vi "ParallelDHT22andBMP180.vi"() -> ()   [LabVIEW 2016]
uses:
  <vilib>/userdefined/High Color/nirio_resource_hc.ctl
  <vilib>/FPGAPlugInAG/myRIO-1900/niLvFpga_Open_myRIO-1900.vi
  <vilib>/FPGAPlugInAG/myRIO-1900/niLvFpga_Run_myRIO-1900.vi
  <vilib>/Utility/error.llb/Error Cluster From Error Code.vi
  <vilib>/rvi/errors/niLvFpgaAdjustHostInterfaceError.vi
  <vilib>/FPGAPlugInAG/myRIO-1900/niLvFpga_Close_myRIO-1900.vi
  <vilib>/rvi/interface/nirviOpenFPGA/nirviOpenFPGA.xnode
  FPGA Bitfiles/WeatherStationPr_FPGATarget_HumiditySensorIn_HuBObqjwKeQ.lvbitx
  <vilib>/rvi/interface/nirviMethod/nirviMethod.xnode
  <vilib>/rvi/interface/nirviReadWriteControl/nirviReadWriteControl.xnode
  <vilib>/rvi/interface/nirviCloseFPGA/nirviCloseFPGA.xnode
  NiFpgaLv.dll
panel:
  in  "stop":bool
  out "Device_ID 2":u8[](array[numeric]) format="%.0x"
  out "READ MSB CAL_PARAM 2":u8[][](array[numeric]) format="%.0x"
  out "READ LSB CAL_PARAM 2":u8[][](array[numeric]) format="%.0x"
  out "Array 3":i16[][](array[numeric])
  out "UP_Value":u16[](array[numeric])
  out "UT_Value 2":u16[](array[numeric])
  out "Temperature(°C)":dbl
  out "Pressure in Pa.":dbl
  out "Waveform Chart Temperature":dbl(graph)
  out "Waveform Chart Presssure":dbl(graph)
  out "error out 2":errorcluster
  out "Waveform Chart":cluster{dbl, dbl}(graph)
  out "Temperature (°C)":fxp<+,16,7> format="%#_3g"
  out "Humidity (%)":fxp<+/-,18,8> format="%#_3g"
  out "Humidity sensor Communication":errorcluster
  out "FPGA Error":errorcluster
  in  "stop 2":bool
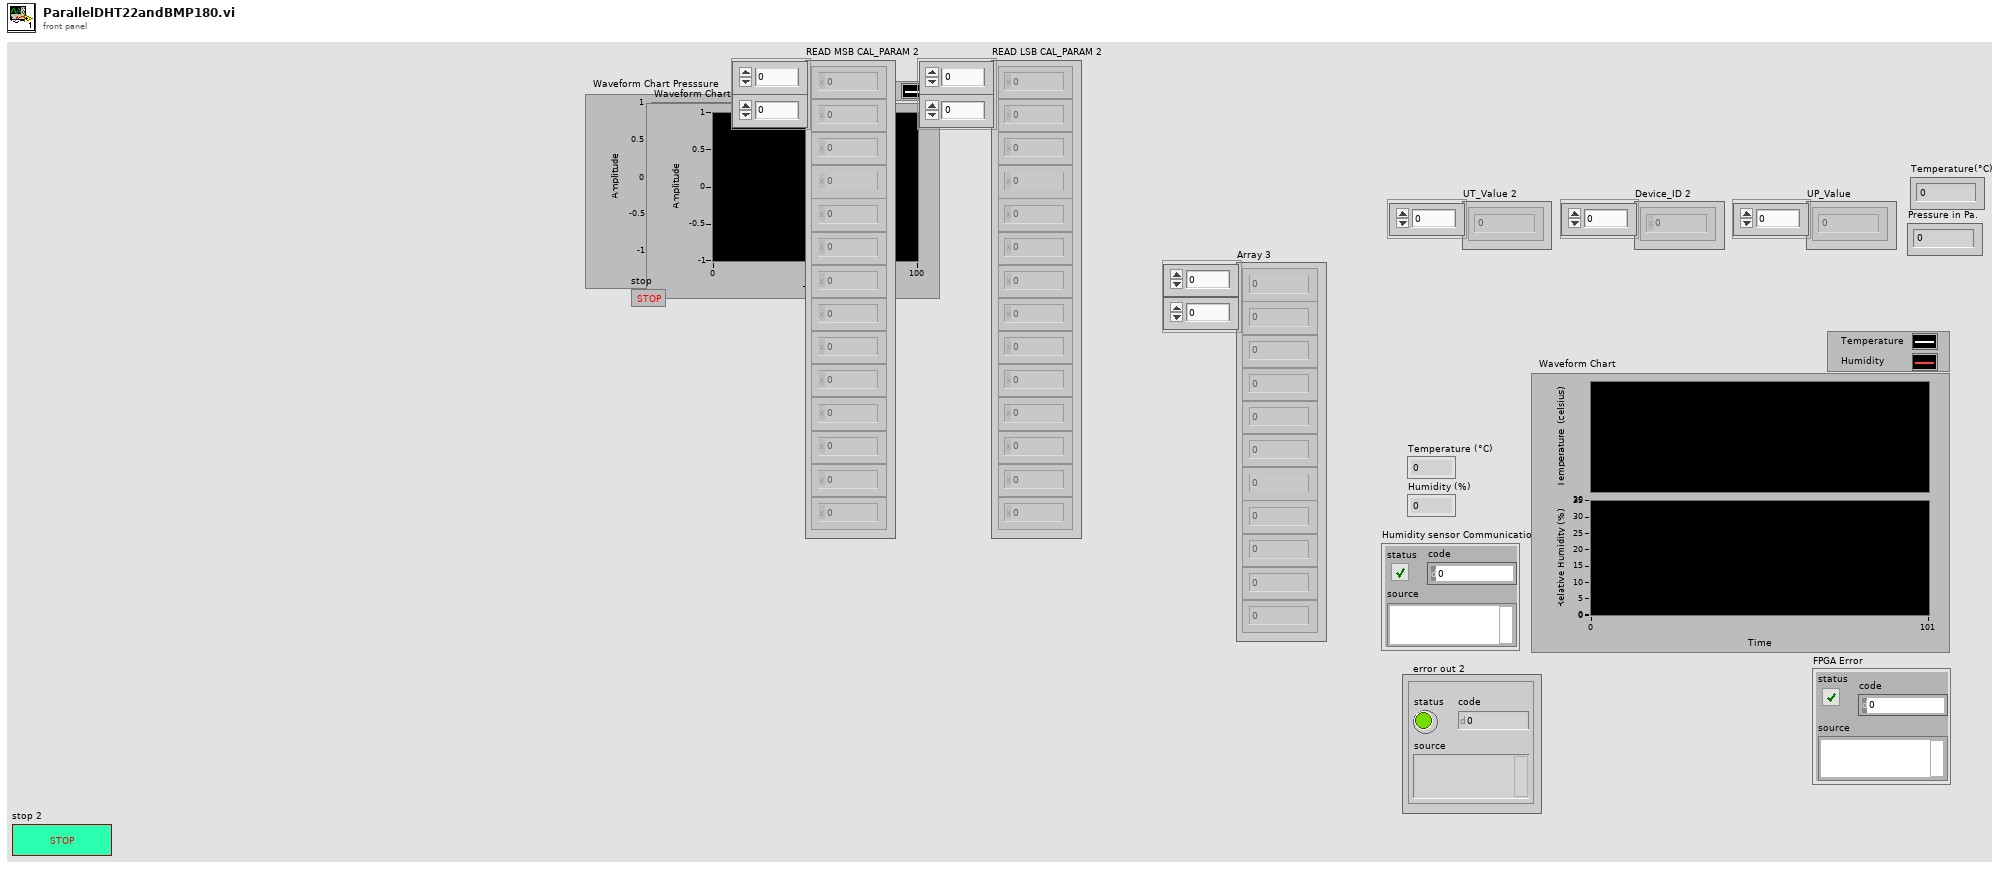
[diagram p1: front panel]
types:
  T1 = typedef "nirio_resource_hc.ctl" = tag
  T2 = cluster{"Temperature (°C)":fxp<+,16,7>, "Humidity (%)":fxp<+/-,18,8>}
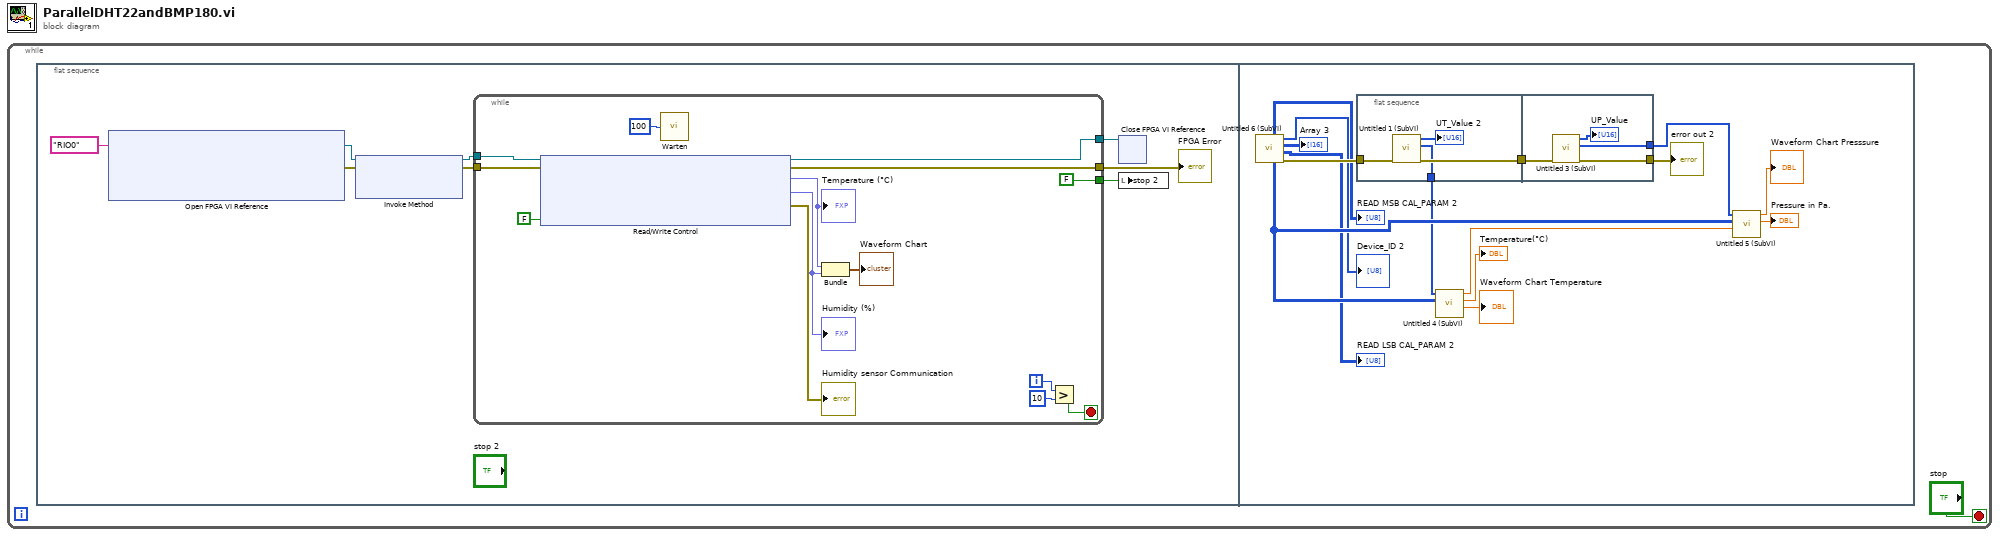
[diagram p0: block diagram]
diagram:
  n1 = while {
    stop <- "stop" stop-if-true
    n2 = flat-sequence {
      frame #0 {
        n3 = xnode "Open FPGA VI Reference"("resource name"=T1 "RIO0") -> ("FPGA VI Reference Out"=w6:refnum<k20>, "error out"=w5:errorcluster)  [unwired: 1 in]
        n4 = xnode "Invoke Method"("FPGA VI Reference In"=w6, "error in"=w5) -> ("FPGA VI Reference Out"=w4:refnum<k20>, "error out"=w3:errorcluster)  [unwired: 1 in]
        n5 = while {
          tunnel: [w18] -> w9
          tunnel: [w13] -> w2
          tunnel: [FALSE] -> w8
          tunnel: w4 -> [w11]
          tunnel: w3 -> [w10]
          i -> [w17]
          stop <- w15 stop-if-true
          n6 = xnode "Read/Write Control"("FPGA VI Reference In"=w11, "error in"=w10, "STOP Reading Inputs"=FALSE ("Warten bis beendet (F)")) -> ("FPGA VI Reference Out"=w13:refnum<k20>, "error out"=w18:errorcluster, "Temperature (°C)"=w21:fxp<+,16,7>, "Humidity (%)"=w22:fxp<+/-,18,8>, "error out"=→"Humidity sensor Communication":errorcluster)
          "Temperature (°C)" <- w21
          "Humidity (%)" <- w22
          n7 = call "Warten"("Count(mSec)"=u32 100) -> ()  [unwired: 1 out]
          n8 = Bundle("Temperature (°C)"=w21, "Humidity (%)"=w22) -> (→"Waveform Chart":T2)  [unwired: 1 in]
          n9 = Greater?(x=w17, y=u32 10 ("Count(mSec)")) -> (0:w15:bool)
        }
        "FPGA Error" <- w9
        n10 = xnode "Close FPGA VI Reference"("FPGA VI Reference In"=w2) -> ()  [unwired: 1 in, 1 out]
        n11 = local write "stop 2"(w8) -> ()
      }
      frame #1 {
        n12 = call "Untitled 6 (SubVI).vi"() -> ("error out"=w37:errorcluster, "READ LSB CAL_PARAM 2"=→"READ LSB CAL_PARAM 2":u8[][], "Array 3"=→"Array 3":i16[][], "Device_ID 2"=→"Device_ID 2":u8[], "Array"=w36:u16[][], "READ MSB CAL_PARAM 2"=→"READ MSB CAL_PARAM 2":u8[][])  [unwired: 6 in]
        n13 = flat-sequence {
          tunnel: w37 -> [w42]
          tunnel: [w41] -> w38
          tunnel: [w40] -> w30
          tunnel: [w45] -> w35
          tunnel: w38 -> [w46]
          tunnel: [w44] -> w28
          frame #0 {
            n14 = call "Untitled 1 (SubVI).vi"("error in (no error)"=w42) -> ("error out"=w41:errorcluster, "Array"=w40:u16[], "UT_Value 2"=→"UT_Value 2":u16[])  [unwired: 8 in]
          }
          frame #1 {
            n15 = call "Untitled 3 (SubVI).vi"("error in (no error)"=w46) -> ("error out"=w45:errorcluster, "Array"=w44:u16[], "UP_Value"=→"UP_Value":u16[])  [unwired: 8 in]
          }
        }
        n16 = call "Untitled 4 (SubVI).vi"("Array"=w36, "Array 2"=w30) -> ("Waveform Chart"=→"Waveform Chart Temperature":dbl, "Temperature(°C)"=→"Temperature(°C)":dbl, "Numeric"=w29:dbl)  [unwired: 7 in]
        n17 = call "Untitled 5 (SubVI).vi"("Numeric"=w29, "Array"=w36, "Array 2"=w28) -> ("Pressure in Pa."=→"Pressure in Pa.":dbl, "Waveform Chart 2"=→"Waveform Chart Presssure":dbl)  [unwired: 7 in]
        "error out 2" <- w35
      }
    }
  }
